vi "Teleop.vi"(8 "Inputs":T1={"West Coast Drive Dev-ref"={"DevStatus"={"status"=FALSE, "code"=0, "source"=""}, "Motors[]"=[], "Square Inputs"=FALSE, "Max Output"=1.0}, "Driver Gamepad"={"Device"=enum."USB 0"}, "Operator Gamepad"={"Device"=enum."USB 0"}, "Shifting Solenoid 1"={"DevStatus"={"status"=FALSE, "code"=0, "source"=""}, "Pneumatics Control Module"=0, "Forward Solenoid Channel"=enum."Invalid", "Reverse Solenoid Channel"=enum."Invalid"}, "Motors"={"Lift Motor 1"={"DeviceStatus"={"status"=FALSE, "code"=0, "source"=""}, "Type"=enum."PWM", "PWM"={"Controller"=enum."Controller 1", "PWM Channel"=enum."Invalid", "DeadBand"={"Name"="", "maxPositivePwm"=0, "minPositivePwm"=0, "centerPwm"=0, "maxNegativePwm"=0, "minNegativePwm"=0, "angularRange"=0}}, "CAN"={"Device Number"=0, "Control Mode"=enum."Percent VBus", "Semaphore"=refnum, "Max Vout"=12.0, "TalonSRX Control Mode"=enum."Percent VBus"}, "Invert"=FALSE, "TransformRef"=refnum, "InvTransformRef"=refnum}, "Gripper Motor"={"DeviceStatus"={"status"=FALSE, "code"=0, "source"=""}, "Type"=enum."PWM", "PWM"={"Controller"=enum."Controller 1", "PWM Channel"=enum."PWM 0", "DeadBand"={"Name"="", "maxPositivePwm"=0, "minPositivePwm"=0, "centerPwm"=0, "maxNegativePwm"=0, "minNegativePwm"=0, "angularRange"=0}}, "CAN"={"Device Number"=0, "Control Mode"=enum."Percent VBus", "Semaphore"=refnum, "Max Vout"=0.0, "TalonSRX Control Mode"=enum."Percent VBus"}, "Invert"=FALSE, "TransformRef"=refnum, "InvTransformRef"=refnum}, "Lift Motor 2"={"DeviceStatus"={"status"=FALSE, "code"=0, "source"=""}, "Type"=enum."PWM", "PWM"={"Controller"=enum."Controller 1", "PWM Channel"=enum."PWM 0", "DeadBand"={"Name"="", "maxPositivePwm"=0, "minPositivePwm"=0, "centerPwm"=0, "maxNegativePwm"=0, "minNegativePwm"=0, "angularRange"=0}}, "CAN"={"Device Number"=0, "Control Mode"=enum."Percent VBus", "Semaphore"=refnum, "Max Vout"=0.0, "TalonSRX Control Mode"=enum."Percent VBus"}, "Invert"=FALSE, "TransformRef"=refnum, "InvTransformRef"=refnum}}, "Limit Switches"={"SwitchDevRef"={"DevStatus"={"status"=FALSE, "code"=0, "source"=""}, "DIO Channel"=enum."DIO 0", "Controller"=enum."Controller 1", "CntIndex"=enum."Ctr 0", "Normally Closed"=FALSE}, "SwitchDevRef 2"={"DevStatus"={"status"=FALSE, "code"=0, "source"=""}, "DIO Channel"=enum."DIO 0", "Controller"=enum."Controller 1", "CntIndex"=enum."Ctr 0", "Normally Closed"=FALSE}, "SwitchDevRef 3"={"DevStatus"={"status"=FALSE, "code"=0, "source"=""}, "DIO Channel"=enum."DIO 0", "Controller"=enum."Controller 1", "CntIndex"=enum."Ctr 0", "Normally Closed"=FALSE}, "SwitchDevRef 4"={"DevStatus"={"status"=FALSE, "code"=0, "source"=""}, "DIO Channel"=enum."DIO 0", "Controller"=enum."Controller 1", "CntIndex"=enum."Ctr 0", "Normally Closed"=FALSE}}, "Drive Encoders"={"EncoderDevRef"={"DevStatus"={"status"=FALSE, "code"=0, "source"=""}, "EncoderIndex"=enum."Enc 0", "CounterIndex"=enum."Ctr 0", "DistancePerCount"=0.0, "Decoding Type"=enum."1x"}, "EncoderDevRef"={"DevStatus"={"status"=FALSE, "code"=0, "source"=""}, "EncoderIndex"=enum."Enc 0", "CounterIndex"=enum."Ctr 0", "DistancePerCount"=0.0, "Decoding Type"=enum."1x"}}, "Gripper Encoder"={"DevStatus"={"status"=FALSE, "code"=0, "source"=""}, "EncoderIndex"=enum."Invalid", "CounterIndex"=enum."Invalid", "DistancePerCount"=1.0, "Decoding Type"=enum."4x"}, "Lift Potentiometer"={"DevStatus"={"status"=FALSE, "code"=0, "source"=""}, "Controller"=enum."Controller 1", "Analog Channel"=enum."Invalid", "Invert Output"=FALSE}, "Shifting Solenoid 2"={"DevStatus"={"status"=FALSE, "code"=0, "source"=""}, "Pneumatics Control Module"=0, "Forward Solenoid Channel"=enum."Invalid", "Reverse Solenoid Channel"=enum."Invalid"}, "Gyro"={"DevStatus"={"status"=FALSE, "code"=0, "source"=""}, "Analog Module"=enum."Controller 1", "Analog Channel"=enum."AI 1", "Offset"=0.0, "Gain (VoltsPerDegree/Second)"=0.0}}) -> ()   [LabVIEW 2014]
doc: "This VI is called for each TeleOp packet received from the DS where the robot is not disabled. It is often used to read from the joysticks and update I/O or to update setpoints for timed control loops. It should complete and return within 20 milliseconds or it may miss DS packets."
uses:
  SubVI/cluster data.ctl
  <vilib>/Rock Robotics/WPI/RobotDrive/WPI_RobotDriveDevRef.ctl
  <vilib>/Rock Robotics/WPI/MotorControl/WPI_MotorControlDeviceRef.ctl
  <vilib>/Rock Robotics/WPI/MotorControl/WPI_MotorControlType.ctl
  <vilib>/Rock Robotics/SystemInterfaces/Typedef/FPGA_TypedefDigitalModule.ctl
  <vilib>/Rock Robotics/SystemInterfaces/DIO/FPGA_DIOPWMChannel.ctl
  <vilib>/Rock Robotics/WPI/PWM/WPI_PWMDeadband.ctl
  <vilib>/Rock Robotics/WPI/CAN/Jaguar/SubVIs/WPI_CANJaguar_ControlMode.ctl
  <vilib>/Rock Robotics/WPI/CAN/TalonSRX/WPI_CANTalonSRX_APIControlMode.ctl
  <vilib>/Rock Robotics/WPI/PWM/WPI_PWMTransform_ConPane.ctl
  <vilib>/Rock Robotics/WPI/Joystick/WPI_JoystickDevRef.ctl
  <vilib>/Rock Robotics/WPI/Joystick/WPI_JoystickDeviceEnum.ctl
  <vilib>/Rock Robotics/WPI/Solenoid/WPI_SolenoidDevRef.ctl
  <vilib>/Rock Robotics/WPI/Solenoid/WPI_SolenoidChannel.ctl
  <vilib>/Rock Robotics/WPI/Switch/WPI_SwitchDevRef.ctl
  <vilib>/Rock Robotics/SystemInterfaces/DIO/FPGA_DIOChannel.ctl
  <vilib>/Rock Robotics/SystemInterfaces/Counter/FPGA_CounterCtrSystemIndex.ctl
  <vilib>/Rock Robotics/WPI/Encoder/WPI_EncoderDevRef.ctl
  <vilib>/Rock Robotics/SystemInterfaces/Encoder/FPGA_EncoderIdx.ctl
  <vilib>/Rock Robotics/WPI/Encoder/WPI_EncoderType.ctl
  <vilib>/Rock Robotics/WPI/Potentiometer/WPI_PotentiometerDevRef.ctl
  <vilib>/Rock Robotics/SystemInterfaces/Typedef/FPGA_TypedefAnalogModule.ctl
  <vilib>/Rock Robotics/SystemInterfaces/AI/FPGA_AIChannel.ctl
  <vilib>/Rock Robotics/WPI/Gyro/WPI_GyroDevRef.ctl
  <vilib>/Rock Robotics/Network Tables/SD Read Number.vi
  <vilib>/Rock Robotics/Network Tables/SD Write Number.vi
  <vilib>/Rock Robotics/Network Tables/SD Write Numeric Array.vi
  <vilib>/Rock Robotics/WPI/Solenoid/Deprecated/WPI_SolenoidSetBool.vi
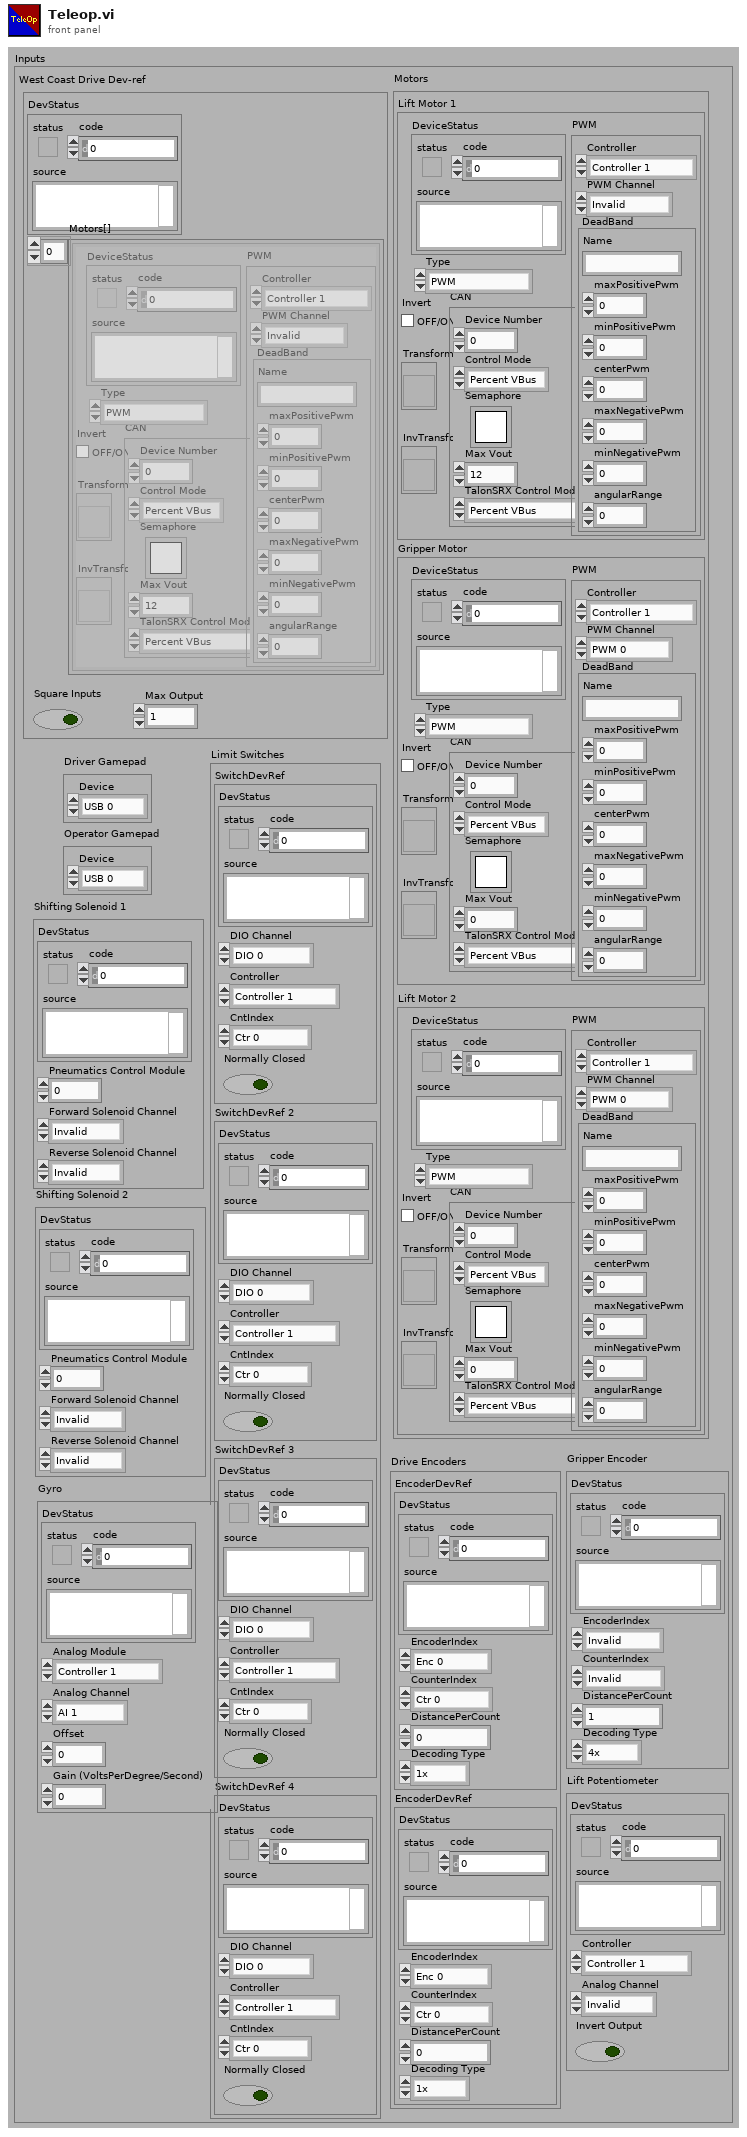
[diagram p1: front panel]
types:
  T1 = typedef "cluster data.ctl" = cluster{"West Coast Drive Dev-ref":T2, "Driver Gamepad":T12, "Operator Gamepad":T12, "Shifting Solenoid 1":T14, "Motors":cluster{"Lift Motor 1":T3, "Gripper Motor":T3, "Lift Motor 2":T3}, "Limit Switches":cluster{"SwitchDevRef":T16, "SwitchDevRef 2":T16, "SwitchDevRef 3":T16, "SwitchDevRef 4":T16}, "Drive Encoders":cluster{"EncoderDevRef":T19, "EncoderDevRef":T19}, "Gripper Encoder":T19, "Lift Potentiometer":T22, "Shifting Solenoid 2":T14, "Gyro":T25}
  T2 = typedef "WPI_RobotDriveDevRef.ctl" = cluster{"DevStatus":errorcluster, "Motors[]":T3[], "Square Inputs":bool, "Max Output":dbl}
  T3 = typedef "WPI_MotorControlDeviceRef.ctl" = cluster{"DeviceStatus":errorcluster, "Type":T4, "PWM":cluster{"Controller":T5, "PWM Channel":T6, "DeadBand":T7}, "CAN":cluster{"Device Number":u8, "Control Mode":T8, "Semaphore":T9, "Max Vout":dbl, "TalonSRX Control Mode":T10}, "Invert":bool, "TransformRef":T11, "InvTransformRef":T11}
  T4 = typedef "WPI_MotorControlType.ctl" = enum16{"PWM", "CAN", "CANTalonSRX"}
  T5 = typedef "FPGA_TypedefDigitalModule.ctl" = enum16{"Controller 1"}
  T6 = typedef "FPGA_DIOPWMChannel.ctl" = enum8{"PWM 0", "PWM 1", "PWM 2", "PWM 3", "PWM 4", "PWM 5", "PWM 6", "PWM 7", "PWM 8", "PWM 9", "PWM MXP 0", "PWM MXP 1", "PWM MXP 2", "PWM MXP 3", "PWM MXP 4", "PWM MXP 5", "PWM MXP 6", "PWM MXP 7", "PWM MXP 8", "PWM MXP 9", "Invalid"}
  T7 = typedef "WPI_PWMDeadband.ctl" = cluster{"Name":string, "maxPositivePwm":i32, "minPositivePwm":i32, "centerPwm":i32, "maxNegativePwm":i32, "minNegativePwm":i32, "angularRange":u16}
  T8 = typedef "WPI_CANJaguar_ControlMode.ctl" = enum8{"Percent VBus", "Current", "Speed", "Position", "Voltage"}
  T9 = typedef "Semaphore RefNum" = refnum<k1>
  T10 = typedef "WPI_CANTalonSRX_APIControlMode.ctl" = enum8{"Percent VBus", "Speed", "Position", "Slave", "Unchanged / Invalid"}
  T11 = typedef "WPI_PWMTransform_ConPane.ctl" = refnum<vi>
  T12 = typedef "WPI_JoystickDevRef.ctl" = cluster{"Device":T13}
  T13 = typedef "WPI_JoystickDeviceEnum.ctl" = enum16{"USB 0", "USB 1", "USB 2", "USB 3", "USB 4", "USB 5"}
  T14 = typedef "WPI_SolenoidDevRef.ctl" = cluster{"DevStatus":errorcluster, "Pneumatics Control Module":u8, "Forward Solenoid Channel":T15, "Reverse Solenoid Channel":T15}
  T15 = typedef "WPI_SolenoidChannel.ctl" = enum8{"Solenoid 0", "Solenoid 1", "Solenoid 2", "Solenoid 3", "Solenoid 4", "Solenoid 5", "Solenoid 6", "Solenoid 7", "Invalid"}
  T16 = typedef "WPI_SwitchDevRef.ctl" = cluster{"DevStatus":errorcluster, "DIO Channel":T17, "Controller":T5, "CntIndex":T18, "Normally Closed":bool}
  T17 = typedef "FPGA_DIOChannel.ctl" = enum8{"DIO 0", "DIO 1", "DIO 2", "DIO 3", "DIO 4", "DIO 5", "DIO 6", "DIO 7", "DIO 8", "DIO 9", "DIO MXP 0", "DIO MXP 1", "DIO MXP 2", "DIO MXP 3", "DIO MXP 4", "DIO MXP 5", "DIO MXP 6", "DIO MXP 7", "DIO MXP 8", "DIO MXP 9", "DIO MXP 10", "DIO MXP 11", "DIO MXP 12", "DIO MXP 13", "DIO MXP 14", "DIO MXP 15", "Invalid"}
  T18 = typedef "FPGA_CounterCtrSystemIndex.ctl" = enum8{"Ctr 0", "Ctr 1", "Ctr 2", "Ctr 3", "Ctr 4", "Ctr 5", "Ctr 6", "Ctr 7", "Invalid"}
  T19 = typedef "WPI_EncoderDevRef.ctl" = cluster{"DevStatus":errorcluster, "EncoderIndex":T20, "CounterIndex":T18, "DistancePerCount":dbl, "Decoding Type":T21}
  T20 = typedef "FPGA_EncoderIdx.ctl" = enum8{"Enc 0", "Enc 1", "Enc 2", "Enc 3", "Enc 4", "Enc 5", "Enc 6", "Enc 7", "Invalid"}
  T21 = typedef "WPI_EncoderType.ctl" = enum16{"1x", "2x", "4x"}
  T22 = typedef "WPI_PotentiometerDevRef.ctl" = cluster{"DevStatus":errorcluster, "Controller":T23, "Analog Channel":T24, "Invert Output":bool}
  T23 = typedef "FPGA_TypedefAnalogModule.ctl" = enum16{"Controller 1"}
  T24 = typedef "FPGA_AIChannel.ctl" = enum8{"AI 0", "AI 1", "AI 2", "AI 3", "AI MXP 0", "AI MXP 1", "AI MXP 2", "AI MXP 3", "Invalid"}
  T25 = typedef "WPI_GyroDevRef.ctl" = cluster{"DevStatus":errorcluster, "Analog Module":T23, "Analog Channel":T24, "Offset":dbl, "Gain (VoltsPerDegree/Second)":dbl}
  T26 = cluster{"Lift Motor 1":T3, "Gripper Motor":T3, "Lift Motor 2":T3}
  T27 = cluster{"EncoderDevRef":T19, "EncoderDevRef":T19}
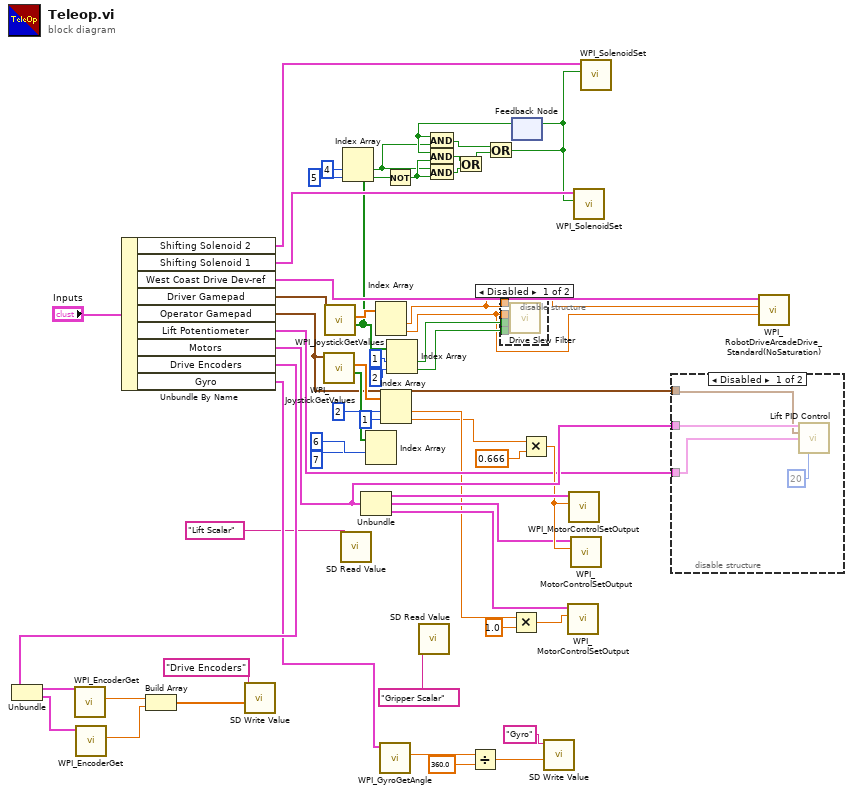
[diagram p0: block diagram]
diagram:
  n1 = Unbundle By Name("Inputs") -> ("Shifting Solenoid 2"=w51:T14, "Shifting Solenoid 1"=w50:T14, "West Coast Drive Dev-ref"=w55:T2, "Driver Gamepad"=w19:T12, "Operator Gamepad"=w1:T12, "Lift Potentiometer"=w32:T22, "Motors"=w34:T26, "Drive Encoders"=w37:T27, "Gyro"=w26:T25)
  n2 = Unbundle(w37) -> ("EncoderDevRef"=w36:T19, "EncoderDevRef"=w35:T19)
  n3 = call <vilib>:"WPI_EncoderGet.vi"("EncoderDevRef"=w36) -> ("Distance"=w30:dbl)  [unwired: 5 in, 5 out]
  n4 = call <vilib>:"WPI_EncoderGet.vi"("EncoderDevRef"=w35) -> ("Distance"=w29:dbl)  [unwired: 5 in, 5 out]
  n5 = Build Array(w30, w29) -> (w28:dbl[])
  n6 = call-poly <vilib>:"SD Write Value.vi"("Numeric Array"=w28, "Name"="Drive Encoders") -> ()  [unwired: 8 in, 2 out]
  n7 = call <vilib>:"WPI_JoystickGetValues.vi"("JoystickDevRef"=w1) -> ("Buttons"=w54:bool[], "Axes"=w11:dbl[])  [unwired: 6 in, 3 out]
  n8 = call <vilib>:"WPI_JoystickGetValues.vi"("JoystickDevRef"=w19) -> ("Buttons"=w6:bool[], "Axes"=w18:dbl[])  [unwired: 6 in, 3 out]
  n9 = call-poly <vilib>:"SD Read Value.vi"("Name"="Lift Scalar") -> ()  [unwired: 8 in, 3 out]
  n10 = Index Array(array=w6, index #1=4 ("index"), index #2=5 ("index")) -> (element #1=w46:bool, element #2=w49:bool)
  n11 = Unbundle(w34) -> ("Lift Motor 1"=w38:T3, "Gripper Motor"=w12:T3, "Lift Motor 2"=w13:T3)
  n12 = Index Array(array=w54, index #1=6 ("index"), index #2=7 ("index")) -> ()  [unwired: 2 out]
  n13 = Index Array(array=w18) -> (element #1=w7:dbl, element #2=w8:dbl)  [unwired: 2 in]
  n14 = call <vilib>:"WPI_GyroGetAngle.vi"("GyroDevRef"=w26) -> ("Angle"=w23:dbl)  [unwired: 7 in, 3 out]
  n15 = Index Array(array=w11, index #1=2 ("index"), index #2=1 ("index")) -> (element #1=w10:dbl, element #2=w2:dbl)
  n16 = Not(x=w49) -> (.not. x?=w48:bool)
  n17 = Index Array(array=w6, index #1=1 ("index"), index #2=2 ("index")) -> (element #1=w15:bool, element #2=w14:bool)
  n18 = call-poly <vilib>:"SD Read Value.vi"("Name"="Gripper Scalar") -> ()  [unwired: 8 in, 3 out]
  n19 = And(x=w46, y=w48) -> (x .and. y?=w44:bool)
  n20 = Divide(x=w23, y=360.0) -> (x/y=w25:dbl)
  n21 = disable-structure shown="Disabled" {
    disable-tunnel: w15 -> [w60 _]
    disable-tunnel: w14 -> [w59 _]
    disable-tunnel: w8 -> [w58 _]
    disable-tunnel: w7 -> [w57 _]
    frame Disabled {
      n22 = call "Drive Slew Filter.vi"("Slew Rate Filter Active?"=w59, "Precision Button"=w60, "Y Axis"=w58, "X Axis"=w57) -> ()  [unwired: 6 in, 2 out]
    }
    frame Enabled {
    }
  }
  n23 = Multiply(x=w10, y=1.0) -> (x*y=w31:dbl)
  n24 = feedback #1() -> (w47:bool)  [unwired: 1 in]
  n25 = And(x=w47, y=w46) -> (x .and. y?=w41:bool)
  n26 = And(x=w47, y=w48) -> (x .and. y?=w45:bool)
  n27 = Or(x=w45, y=w44) -> (x .or. y?=w43:bool)
  n28 = Or(x=w41, y=w43) -> (x .or. y?=w42:bool)
  n29 = feedback-in #1(w42) -> ()
  n30 = Multiply(x=w2, y=0.666) -> (x*y=w33:dbl)
  n31 = call-poly <vilib>:"SD Write Value.vi"("Numeric"=w25, "Name"="Gyro" ("Table Prefix")) -> ()  [unwired: 8 in, 2 out]
  n32 = call <vilib>:"WPI_MotorControlSetOutput.vi"("Output"=w31, "MotorControlDevRef"=w13) -> ()  [unwired: 7 in, 3 out]
  n33 = call <vilib>:"WPI_MotorControlSetOutput.vi"("Output"=w33, "MotorControlDevRef"=w38) -> ()  [unwired: 7 in, 3 out]
  n34 = call <vilib>:"WPI_MotorControlSetOutput.vi"("Output"=w33, "MotorControlDevRef"=w12) -> ()  [unwired: 7 in, 3 out]
  n35 = call-poly <vilib>:"WPI_SolenoidSet.vi"("Value"=w42, "SolenoidDevRef"=w50) -> ()  [unwired: 8 in, 2 out]
  n36 = call-poly <vilib>:"WPI_SolenoidSet.vi"("Value"=w42, "SolenoidDevRef"=w51) -> ()  [unwired: 8 in, 2 out]
  n37 = disable-structure shown="Disabled" {
    disable-tunnel: w34 -> [w64 _]
    disable-tunnel: w32 -> [w61 _]
    disable-tunnel: w1 -> [w62 _]
    frame Disabled {
      n38 = call "Lift PID Control.vi"("Motor DevRefs IN"=w64, "Operator Gamepad"=w62, "Lift Potentionmeter"=w61, "Time to Wait"=20) -> ()  [unwired: 10 in, 2 out]
    }
    frame Enabled {
    }
  }
  n39 = call <vilib>:"WPI_RobotDriveArcadeDrive_Standard(NoSaturation).vi"("Y axis value"=w8, "X axis value"=w7, "RobotDriveDevRef"=w55) -> ()  [unwired: 1 in, 8 out]
